vi "Simple Read.vi"(4 "Class":refnum<class "Abs_Complex Extended Float.lvclass">) -> (1 "Value":cxt)   [LabVIEW 2021, in "Abs_Complex Extended Float.lvclass"]
uses:
  Abs_Complex Extended Float.lvclass
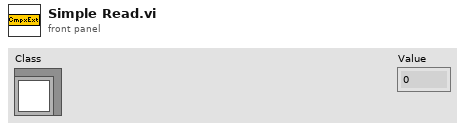
[diagram p1: front panel]
types:
  T1 = typedef "Abs_Complex Extended Float.lvclass/Type.ctl" = cxt
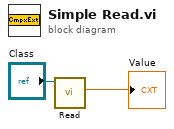
[diagram p0: block diagram]
diagram:
  n1 = call-dynamic "Read.vi"("Double Float.lvclass_340760 in"="Class") -> ("Value"=→"Value":T1)  [unwired: 8 in, 2 out]
